vi "Actor Receive.vi"(11 "Dev Actor in":refnum<class "Dev Actor.lvclass">) -> (2 "Msg":refnum<class "Msg Strategy.lvclass">, 3 "Dev Actor out":refnum<class "Dev Actor.lvclass">)   [LabVIEW 2021, in "Dev Actor.lvlib" / "Dev Actor.lvclass"]
uses:
  Dev Actor.lvclass
  <vilib>/jettl/jettl/jettl/Msg Strategy/Msg Strategy.lvclass
  Dev Actor.lvclass/Dev Actor.ctl
  <vilib>/jettl/jettl/jettl/Actor/Actor.lvclass
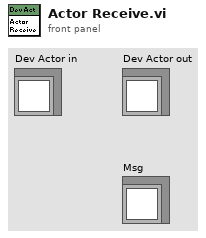
[diagram p1: front panel]
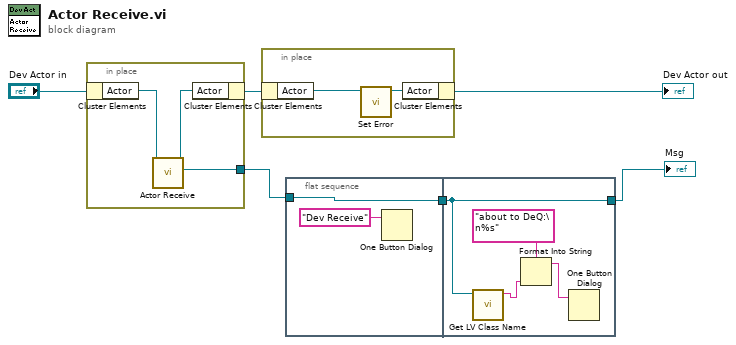
[diagram p0: block diagram]
diagram:
  n1 = in-place {
    in-place-border: [w7] -> w2
    n2 = in-place-cluster #1("Dev Actor in") -> ("Actor"=w9:refnum<class "Actor.lvclass">)
    n3 = call-dynamic "Actor Receive.vi"("Actor in"=w9) -> ("Msg"=w7:refnum<class "Msg Strategy.lvclass">, "Actor out"=w8:refnum<class "Actor.lvclass">)  [unwired: 9 in]
    n4 = in-place-cluster #1("Actor"=w8) -> (w5:refnum<class "Dev Actor.lvclass">)
  }
  n5 = in-place {
    n6 = in-place-cluster #2(w5) -> ("Actor"=w11:refnum<class "Actor.lvclass">)
    n7 = call-dynamic "Set Error.vi"("Actor in"=w11) -> ("Actor out"=w10:refnum<class "Actor.lvclass">)  [unwired: 10 in]
    n8 = in-place-cluster #2("Actor"=w10) -> (→"Dev Actor out":refnum<class "Dev Actor.lvclass">)
  }
  n9 = flat-sequence {
    tunnel: [w12] -> w3
    tunnel: w2 -> [w12]
    tunnel: [w17] -> w1
    tunnel: w3 -> [w17]
    frame #0 {
      n10 = One Button Dialog(message="Dev Receive") -> ()  [unwired: 1 in, 1 out]
    }
    frame #1 {
      n11 = call <vilib>:"Get LV Class Name.vi"("object"=w17) -> ("class name"=w16:string)  [unwired: 9 in, 1 out]
      n12 = Format Into String(format string="about to DeQ:\n%s", w16) -> (resulting string=w15:string)  [unwired: 2 in, 1 out]
      n13 = One Button Dialog(message=w15) -> ()  [unwired: 1 in, 1 out]
    }
  }
  "Msg" <- w1
